vi "Retreive Project Root Ref.vi"(8 "error in (no error)":errorcluster, 11 "Project in":refnum<vi>) -> (0 "error out":errorcluster, 2 "Project Root out":refnum<vi>, 3 "Project out":refnum<vi>)   [LabVIEW 2019, in "Project Sync Tools.lvclass"]
uses:
  Project Sync Tools.lvclass
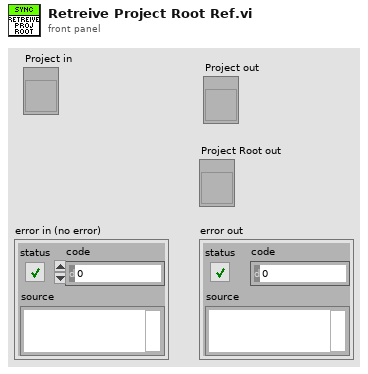
[diagram p1: front panel]
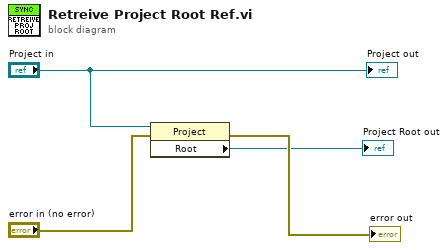
[diagram p0: block diagram]
diagram:
  n1 = property class="Project"(reference="Project in", error in="error in (no error)") -> (error out=→"error out":errorcluster, "Root"=→"Project Root out":refnum<vi>)  [unwired: 1 out]
  "Project out" <- "Project in"
